vi "区域曲线.vi"(8 "区域最大压力(N)":dbl, 9 "区域最小压力(N)":dbl, 10 "区域最大位移(mm)":dbl, 11 "区域最小位移(mm)":dbl) -> (2 "区域曲线":cluster{dbl[], dbl[]}(graph) caption="压球涨堵头1")   [LabVIEW 2013]
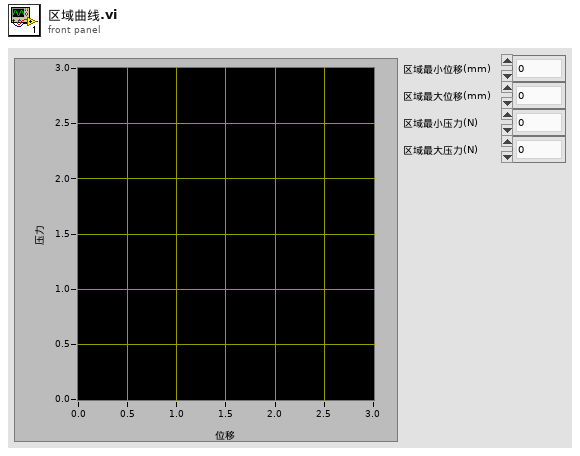
[diagram p1: front panel]
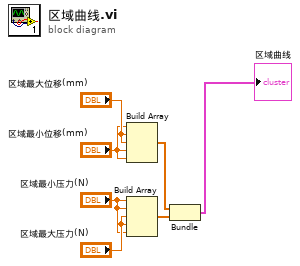
[diagram p0: block diagram]
diagram:
  n1 = Build Array("区域最小位移(mm)", "区域最大位移(mm)", "区域最大位移(mm)", "区域最小位移(mm)", "区域最小位移(mm)") -> (w2:dbl[])
  n2 = Build Array("区域最小压力(N)", "区域最小压力(N)", "区域最大压力(N)", "区域最大压力(N)", "区域最小压力(N)") -> (w3:dbl[])
  n3 = Bundle(w2, w3) -> (→"区域曲线":cluster{dbl[], dbl[]})  [unwired: 1 in]
